vi "TreeAdminSetNoOfTrials(SubVI).vi"() -> ()   [LabVIEW 2013]
uses:
  FYP_LabviewGlobal(SubVI).vi
panel:
  out "Active Cell:String":string
  out "Get Theme Admin":string
  out "Get Topic Admin":string
  out "Get Paper Admin":string
  in  "LogOut":bool
  in  "Tree 4":string(tree)
  # "Please select one Paper First"
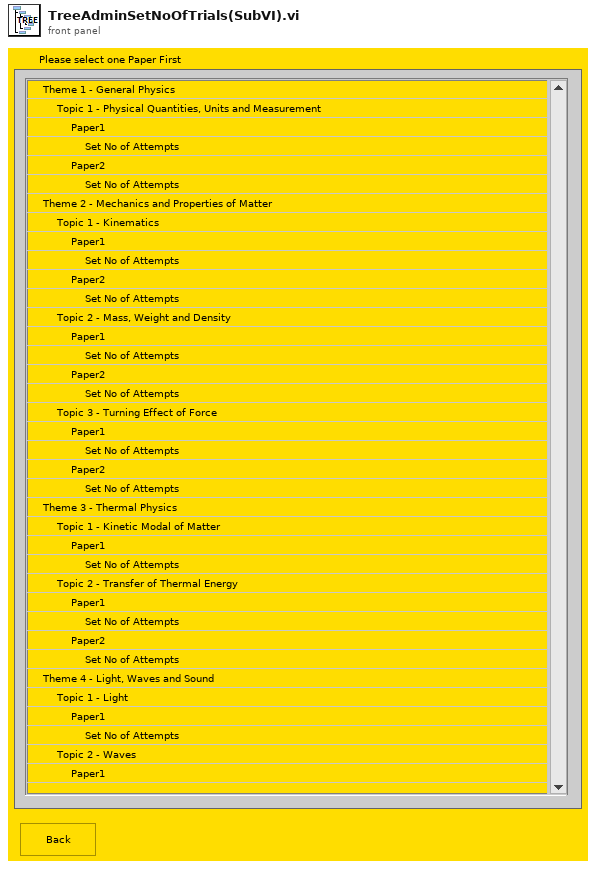
[diagram p1: front panel]
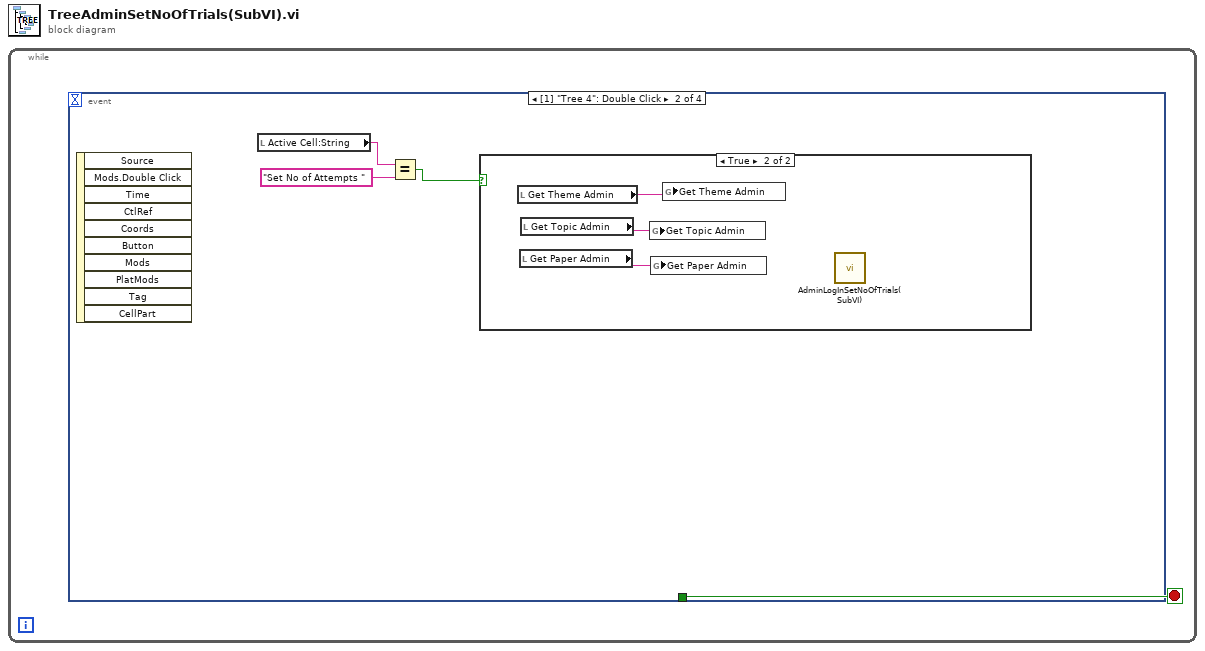
[diagram p0: block diagram]
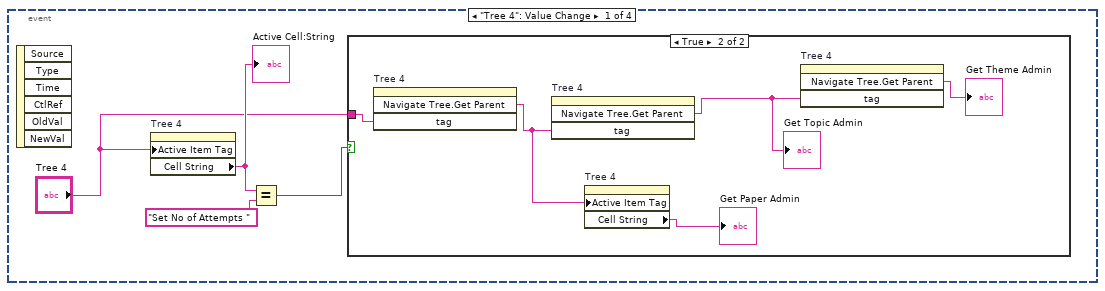
[diagram p2: hidden frame]
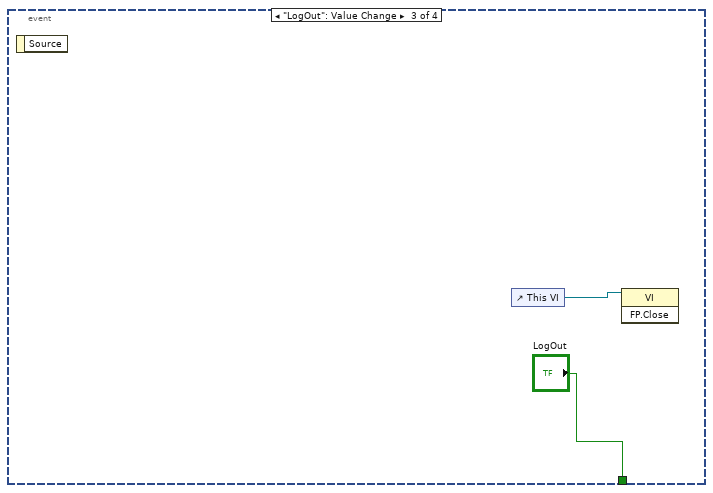
[diagram p5: hidden frame]
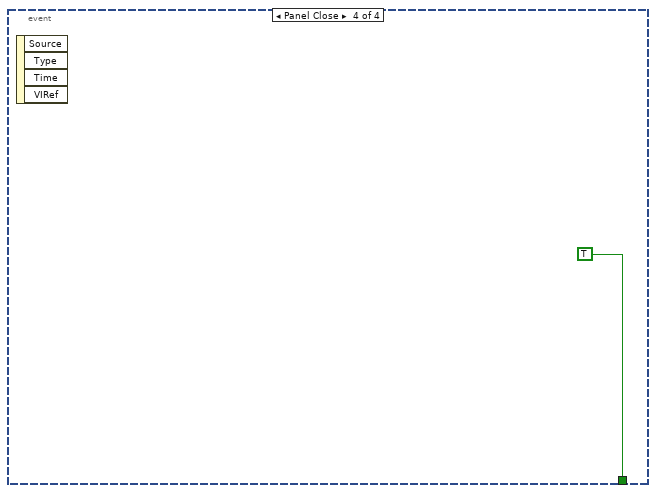
[diagram p6: hidden frame]
diagram:
  n1 = while {
    stop <- w1 stop-if-true
    n2 = event shown="[1] \"Tree 4\": Double Click" {
      selector: _ -> [_ _ _ _]
      dyn-events: _ -> [_ _ _ _]
      timeout: _ -> [_ _ _ _]
      tunnel: [_ _ "LogOut" TRUE] -> w1
      event "Tree 4": Value Change {
        n3 = event-data() -> ()  [unwired: 1 in, 6 out]
        n4 = property on="Tree 4" class="Tree (strict)"("Active Item Tag"="Tree 4") -> ("Cell String"=w4:string)  [unwired: 2 in, 2 out]
        "Active Cell:String" <- w4
        n5 = Equal?(x=w4, y="Set No of Attempts ") -> (x = y?=w3:bool)
        n6 = case shown="True" w3 {
          tunnel: "Tree 4" -> [_ w6]
          frame False {
          }
          frame True {
            n7 = invoke on="Tree 4" class="Tree (strict)" method="Navigate Tree.Get Parent"("tag"=w6) -> ("Navigate Tree:Get Parent"=w10:string)  [unwired: 3 in, 3 out]
            n8 = invoke on="Tree 4" class="Tree (strict)" method="Navigate Tree.Get Parent"("tag"=w10) -> ("Navigate Tree:Get Parent"=w8:string)  [unwired: 3 in, 3 out]
            "Get Topic Admin" <- w8
            n9 = property on="Tree 4" class="Tree (strict)"("Active Item Tag"=w10) -> ("Cell String"=→"Get Paper Admin":string)  [unwired: 2 in, 2 out]
            n10 = invoke on="Tree 4" class="Tree (strict)" method="Navigate Tree.Get Parent"("tag"=w8) -> ("Navigate Tree:Get Parent"=→"Get Theme Admin":string)  [unwired: 3 in, 3 out]
          }
        }
      }
      event "Tree 4": Double Click {
        n11 = event-data() -> ()  [unwired: 1 in, 10 out]
        n12 = local read "Active Cell:String"() -> (w13:string)
        n13 = Equal?(x=w13, y="Set No of Attempts ") -> (x = y?=w11:bool)
        n14 = case shown="True" w11 {
          frame False {
          }
          frame True {
            n15 = local read "Get Theme Admin"() -> (w16:string)
            n16 = local read "Get Paper Admin"() -> (w14:string)
            n17 = local read "Get Topic Admin"() -> (w15:string)
            n18 = global write "FYP_LabviewGlobal(SubVI).vi" "Get Topic Admin"(w15) -> ()
            n19 = global write "FYP_LabviewGlobal(SubVI).vi" "Get Paper Admin"(w14) -> ()
            n20 = global write "FYP_LabviewGlobal(SubVI).vi" "Get Theme Admin"(w16) -> ()
            n21 = call "AdminLogInSetNoOfTrials(SubVI).vi"() -> ()  [unwired: 12 in]
          }
        }
      }
      event "LogOut": Value Change {
        n22 = event-data() -> ()  [unwired: 1 in, 1 out]
        n23 = control-ref of="This VI"() -> (w18:refnum<vi>)
        n24 = invoke class="VI" method="FP.Close"(reference=w18) -> ()  [unwired: 2 in, 3 out]
      }
      event Panel Close {
        n25 = event-data() -> ()  [unwired: 1 in, 4 out]
      }
    }
  }
